vi "Get actuator info.vi"(8 "error in (no error)":errorcluster, 11 "VISA Refnum in":refnum<visa-resource-name>) -> (0 "error out":errorcluster, 2 "String":string, 3 "Array":string[](array[string]))   [LabVIEW 2016]
uses:
  Controls/Command list.ctl
  Controls/Command cluster.ctl
panel:
  out "Array 2":string[](array[string])
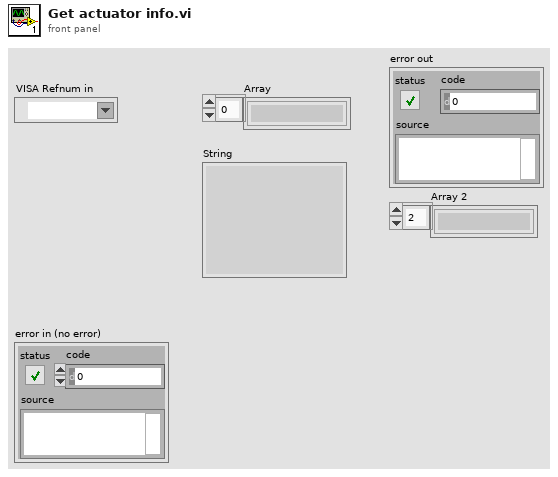
[diagram p1: front panel]
types:
  T1 = typedef "Command cluster.ctl" = cluster{"Command":T2, "data":variant}
  T2 = typedef "Command list.ctl" = enum16{"", "£nabort", "getaxisno", "£getserialno", "£nidentify", "&&£setnlimit", "&£nm", "&£snv", "&£speed", "£np", "£ncal"}
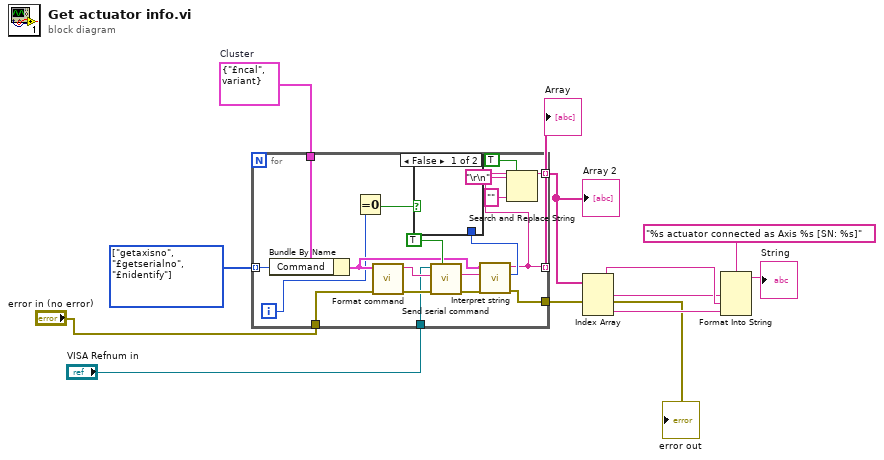
[diagram p0: block diagram]
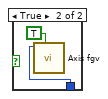
[diagram p2: hidden frame]
diagram:
  w2 = T1 {"Command"=enum."£ncal", "data"=variant}  # Cluster
  w4 = T2[] [enum."getaxisno", enum."£getserialno", enum."£nidentify"] items=["", "£nabort", "getaxisno", "£getserialno", "£nidentify", "&&£setnlimit", "&£nm", "&£snv", "&£speed", "£np", "£ncal"]
  n1 = for {
    tunnel: w2 -> [w31]
    tunnel: w4 -> [w30] mode=indexing
    tunnel: "error in (no error)" -> [w29]
    tunnel: "VISA Refnum in" -> [w26]
    tunnel: [w17] -> w7 mode=indexing
    tunnel: [w21] -> w3
    tunnel: [w14] -> w1 mode=indexing
    i -> [w20]
    n2 = Bundle By Name(cluster=w31, "Command"=w30) -> (w23:T1)
    n3 = Equal To 0?(x=w20) -> (x = 0?=w19:bool)
    n4 = call "Format command.vi"("error in (no error)"=w29, "Cluster"=w23) -> ("error out"=w28:errorcluster, "String"=w27:string)  [unwired: 8 in]
    n5 = call "Send serial command.vi"("Read?"=TRUE, "error IO"=w28, "Send string"=w27, "VISA resource name out"=w26) -> ("error out"=w24:errorcluster, "read string"=w22:string)  [unwired: 5 in, 1 out]
    n6 = call "Interpret string.vi"("error in (no error)"=w24, "String"=w22, "Cluster"=w23) -> ("error out"=w21:errorcluster, "Numeric"=w18:u16, "String 2"=w17:string)  [unwired: 5 in, 1 out]
    n7 = case shown="False" w19 {
      tunnel: w18 -> [_ w32]
      frame False {
      }
      frame True {
        n8 = call "Axis fgv.vi"("Set"=TRUE, "Axis"=w32) -> ()  [unwired: 8 in, 2 out]
      }
    }
    n9 = Search and Replace String(replace all?=TRUE ("replace all? (F)"), input string=w17, search string="\r\n", replace string="" ("replace string (\"\")")) -> (result string=w14:string)  [unwired: 4 in, 3 out]
  }
  "Array" <- w7
  "error out" <- w3
  "Array 2" <- w1
  n10 = Index Array(array=w1) -> (element #1=w11:string, element #2=w12:string, element #3=w10:string)  [unwired: 3 in]
  n11 = Format Into String(format string="%s actuator connected as Axis %s [SN: %s]", w10, w11, w12) -> (resulting string=→"String":string)  [unwired: 2 in, 1 out]
